vi "Configure Output Enabled.vi"(8 "error in (no error)":errorcluster {"code" format="%.0x"}, 9 "Enable Output (False)":bool, 10 "Channel Name (1)":string="1", 11 "VISA resource name":refnum<visa-resource-name>) -> (0 "error out":errorcluster {"code" format="%.0x"}, 3 "VISA resource name out":refnum<visa-resource-name>)   [LabVIEW 2018, in "Agilent N6700 Series.lvlib"]
doc: "Configures whether the signal that the power supply produces on a channel appears at the output connector."
uses:
  Agilent N6700 Series.lvlib
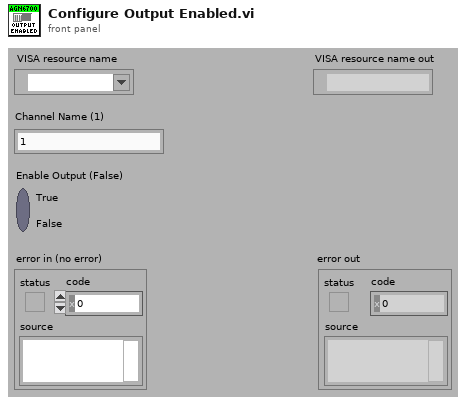
[diagram p1: front panel]
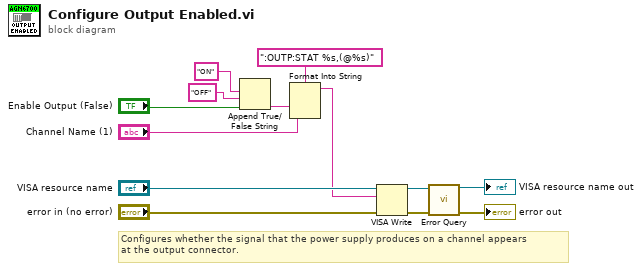
[diagram p0: block diagram]
diagram:
  # "Configures whether the signal that the power supply produces on a channel appears \nat the output connector."
  n1 = Append True/False String(1:"Enable Output (False)", 2:"OFF", 3:"ON") -> (0:w9:string)  [unwired: 1 in]
  n2 = Format Into String(format string=":OUTP:STAT %s,(@%s)", w9, "Channel Name (1)") -> (resulting string=w5:string)  [unwired: 2 in, 1 out]
  n3 = VISA Write(VISA resource name="VISA resource name", write buffer=w5, error in (no error)="error in (no error)") -> (VISA resource name out=w2:refnum<visa-resource-name>, error out=w1:errorcluster)  [unwired: 1 out]
  n4 = call "Error Query.vi"("VISA resource name"=w2, "error in (no error)"=w1) -> ("VISA resource name out"=→"VISA resource name out":refnum<visa-resource-name>, "error out"=→"error out":errorcluster)  [unwired: 10 in, 2 out]
